vi "FFT x(t) to dB,Degrees.vi"   [LabVIEW 2020]
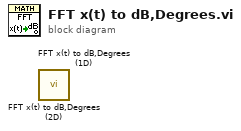
[diagram p0: block diagram]
diagram:
  n1 = call "FFT x(t) to dB,Degrees (2D).vi"() -> ()  [unwired: 9 in, 3 out]
  n2 = call "FFT x(t) to dB,Degrees (1D).vi"() -> ()  [unwired: 9 in, 3 out]
